vi "V001 - Variable DC Controller - With Buttons - Speed Control.vi"() -> ()   [LabVIEW 2022 SP3]
panel:
  in  "Stop Button":bool
  in  "Start Button":bool
  in  "Button 3":bool
  in  "Button 2":bool
  in  "Button 1":bool
  in  "Exit Button":bool
  in  "Connect":bool
  in  "VISA resource name":refnum<visa-resource-name>
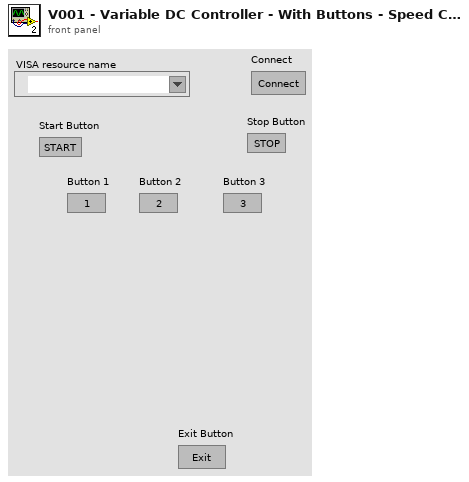
[diagram p1: front panel]
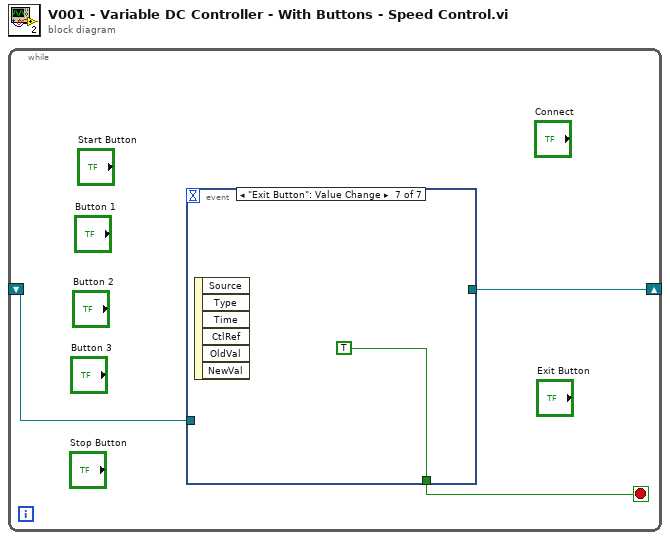
[diagram p0: block diagram]
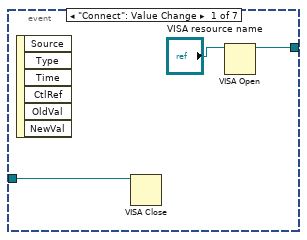
[diagram p2: hidden frame]
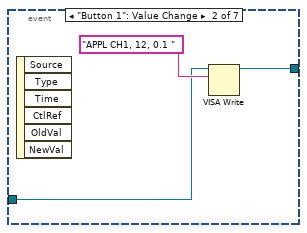
[diagram p3: hidden frame]
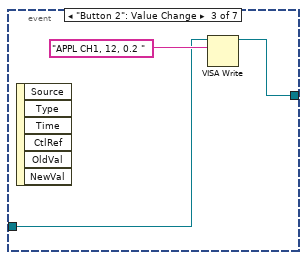
[diagram p4: hidden frame]
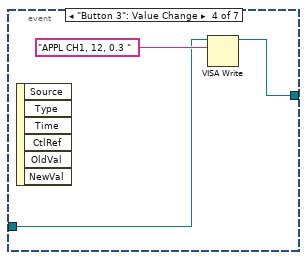
[diagram p5: hidden frame]
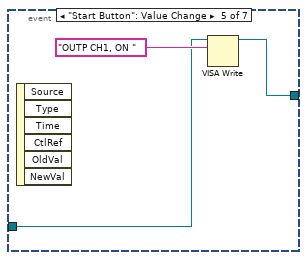
[diagram p6: hidden frame]
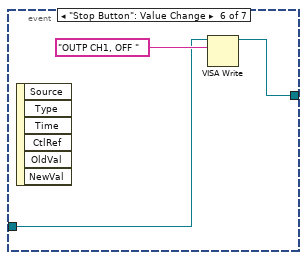
[diagram p7: hidden frame]
diagram:
  n1 = while {
    shift-right: [w3] -> _
    shift-left: _ -> [w2]
    stop <- w1 stop-if-true
    n2 = event shown="[6] \"Exit Button\": Value Change" {
      selector: _ -> [_ _ _ _ _ _ _]
      dyn-events: _ -> [_ _ _ _ _ _ _]
      timeout: _ -> [_ _ _ _ _ _ _]
      tunnel: [w5 w8 w11 w14 w17 w20 _] -> w3
      tunnel: w2 -> [w4 w7 w10 w13 w16 w19 _]
      tunnel: [_ _ _ _ _ _ TRUE] -> w1
      event "Connect": Value Change {
        n3 = event-data() -> ()  [unwired: 1 in, 6 out]
        n4 = VISA Close(VISA resource name=w4) -> ()  [unwired: 1 in, 1 out]
        n5 = VISA Open(VISA resource name="VISA resource name") -> (VISA resource name=w5:refnum<visa-resource-name>)  [unwired: 4 in, 1 out]
      }
      event "Button 1": Value Change {
        n6 = event-data() -> ()  [unwired: 1 in, 6 out]
        n7 = VISA Write(VISA resource name=w7, write buffer="APPL CH1, 12, 0.1 ") -> (VISA resource name out=w8:refnum<visa-resource-name>)  [unwired: 1 in, 2 out]
      }
      event "Button 2": Value Change {
        n8 = event-data() -> ()  [unwired: 1 in, 6 out]
        n9 = VISA Write(VISA resource name=w10, write buffer="APPL CH1, 12, 0.2 ") -> (VISA resource name out=w11:refnum<visa-resource-name>)  [unwired: 1 in, 2 out]
      }
      event "Button 3": Value Change {
        n10 = event-data() -> ()  [unwired: 1 in, 6 out]
        n11 = VISA Write(VISA resource name=w13, write buffer="APPL CH1, 12, 0.3 ") -> (VISA resource name out=w14:refnum<visa-resource-name>)  [unwired: 1 in, 2 out]
      }
      event "Start Button": Value Change {
        n12 = event-data() -> ()  [unwired: 1 in, 6 out]
        n13 = VISA Write(VISA resource name=w16, write buffer="OUTP CH1, ON ") -> (VISA resource name out=w17:refnum<visa-resource-name>)  [unwired: 1 in, 2 out]
      }
      event "Stop Button": Value Change {
        n14 = event-data() -> ()  [unwired: 1 in, 6 out]
        n15 = VISA Write(VISA resource name=w19, write buffer="OUTP CH1, OFF ") -> (VISA resource name out=w20:refnum<visa-resource-name>)  [unwired: 1 in, 2 out]
      }
      event "Exit Button": Value Change {
        n16 = event-data() -> ()  [unwired: 1 in, 6 out]
      }
    }
  }
